vi "Invoke IL Action.vi"(6 "IL Action":refnum<class "IL Action.lvclass">[](array[class]), 8 "error in (no error)":errorcluster, 10 "Caller Enqueuer":refnum<class "Message Enqueuer.lvclass">, 11 "Interlock Chain in":refnum<class "Interlock Chain.lvclass">) -> (0 "error out":errorcluster, 3 "Interlock Chain out":refnum<class "Interlock Chain.lvclass">, 4 "Stop Self?":bool)   [LabVIEW 2015, in "Interlocks.lvlib" / "Interlock Chain.lvclass"]
uses:
  Interlocks/Interlock Chain/Interlock Chain.lvclass
  <vilib>/ActorFramework/Message Enqueuer/Message Enqueuer.lvclass
  Interlocks/IL Action/IL Action.lvclass
  <vilib>/ActorFramework/Stop Msg/Stop Msg.lvclass
  <vilib>/ActorFramework/Message/Message.lvclass
  Interlocks/IL Action/IL Action.lvclass/IL Action.ctl
  <vilib>/ActorFramework/Message Enqueuer/Message Enqueuer.lvclass/Message Enqueuer.ctl
  <vilib>/ActorFramework/Message Priority Queue/Priority Enqueue.vi
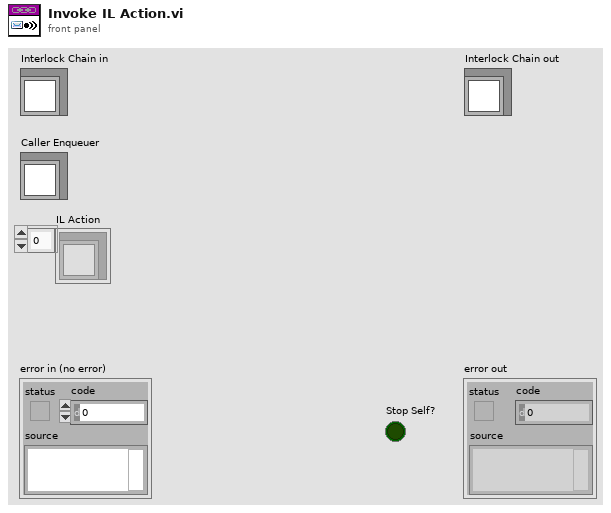
[diagram p1: front panel]
types:
  T1 = typedef "Actor Framework.lvlib/Message Enqueuer.lvclass/Message Priority.ctl" = enum16{"Low", "Normal", "High"}
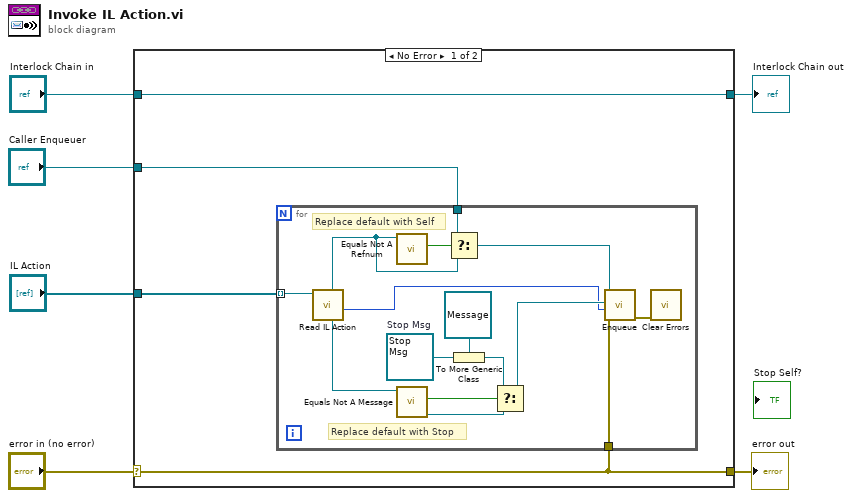
[diagram p0: block diagram]
diagram:
  n1 = case shown="No Error" "error in (no error)" {
    selector: "error in (no error)" -> [w8 w27]
    tunnel: [w8 w27] -> w5
    tunnel: "Caller Enqueuer" -> [w9 _]
    tunnel: "IL Action" -> [w10 _]
    tunnel: "Interlock Chain in" -> [w7 w26]
    tunnel: [w7 w26] -> w1
    frame No Error {
      n2 = for {
        tunnel: w10 -> [w25] mode=indexing
        tunnel: w9 -> [w23]
        tunnel: w8 -> [w12]
        w18 = refnum<class "Stop Msg.lvclass"> refnum  # Stop Msg
        # "Replace default with Stop"
        # "Replace default with Self"
        n3 = call "Read IL Action.vi"("IL Action in"=w25) -> ("Message Priority"=w13:T1, "Actor Framework:Message"=w21:refnum<class "Message.lvclass">, "Action Destination"=w22:refnum<class "Message Enqueuer.lvclass">)  [unwired: 7 in, 1 out]
        n4 = call <vilib>:"Equals Not A Refnum.vi"("Message Enqueuer"=w22) -> ("Not a refnum?"=w24:bool)  [unwired: 10 in]
        n5 = call "Equals Not A Message.vi"("Actor Framework:Message"=w21) -> ("Actor Framework:Message out"=w19:refnum<class "Message.lvclass">, "Not a refnum?"=w20:bool)  [unwired: 9 in]
        n6 = Select(t=w23, s=w24, f=w22) -> (s? t:f=w15:refnum<class "Message Enqueuer.lvclass">)
        n7 = To More Generic Class(target class=refnum<class "Message.lvclass"> refnum ("t"), reference=w18) -> (generic class reference=w17:refnum<class "Message.lvclass">)
        n8 = Select(t=w17, s=w20, f=w19) -> (s? t:f=w14:refnum<class "Message.lvclass">)
        n9 = call <vilib>:"Enqueue.vi"("error in (no error)"=w12, "Message Priority (Normal)"=w13, "Message"=w14, "Message Enqueuer in"=w15) -> ("error out"=w11:errorcluster)  [unwired: 6 in, 1 out]
        n10 = call <vilib>:"Clear Errors.vi"("error in (no error)"=w11) -> ()  [unwired: 5 in, 2 out]
      }
    }
    frame Error {
    }
  }
  "error out" <- w5
  "Interlock Chain out" <- w1
